vi "Vending_Machine.vi"(0 "Rs100":bool, 1 "Coke":bool, 2 "Fanta":bool, 3 "Sprite":bool, 5 "Rs50":bool, 7 "Rs20":bool, 9 "Rs10":bool, 11 "Rs5":bool, 12 "Cancel":bool, 13 "Open_Door":bool, 14 "Reset":bool) -> (4 "Display_Message":string, 6 "Total_Number_of_Cans":i32 caption="Total Number of Cans", 8 "Total_Cash":i32 caption="Total Cash")   [LabVIEW 2021]
doc: "This is the Coke Vending machine."
uses:
  Controls/Queue_Driver_Select.ctl
  Controls/Inserted_Cash_Count.ctl
  Controls/INI_Operation_Select.ctl
  Controls/Timer_Select.ctl
  Controls/Total_Cash_Count.ctl
  Controls/INI_Data.ctl
  Controls/Controls_Referece.ctl
  Controls/Vending_Data.ctl
panel:
  out "Drink_Ready?":bool
  out "Error_Out":errorcluster
  in  "Error_In":errorcluster
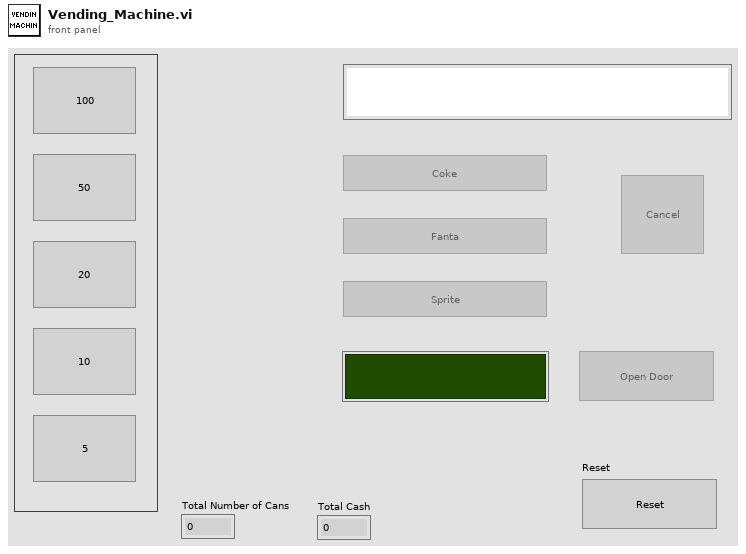
[diagram p1: front panel]
types:
  T1 = typedef "Vending_Data.ctl" = cluster{"INI_Data":T2, "Inserted_Cash_Count":T4, "Drink_Type":string, "Display_Message":string, "Drink_Ready?":bool, "Open_Door":bool, "Cancel":bool, "Reset":bool, "Gray_Out_Control":refnum<vi>[], "Enable_Control":refnum<vi>[], "Disable_Control":refnum<vi>[], "Selected_Cool_Drink":string, "Controls_Reference":T5, "States":string[], "Time_Out":bool, "Exit":bool, "Cost_Per_Can":i32}
  T2 = typedef "INI_Data.ctl" = cluster{"Total_Cash_Count":T3, "Total_Number_of_Cans":i32, "Total_Cash":i32}
  T3 = typedef "Total_Cash_Count.ctl" = cluster{"Rs100":i32, "Rs50":i32, "Rs20":i32, "Rs10":i32, "Rs5":i32}
  T4 = typedef "Inserted_Cash_Count.ctl" = cluster{"Rs100":i32, "Rs50":i32, "Rs20":i32, "Rs10":i32, "Rs5":i32}
  T5 = typedef "Controls_Referece.ctl" = cluster{"Sprite":refnum<vi>, "Fanta":refnum<vi>, "Coke":refnum<vi>, "Cancel":refnum<vi>, "Open_Door":refnum<vi>, "Rs100":refnum<vi>, "Rs50":refnum<vi>, "Rs20":refnum<vi>, "Rs10":refnum<vi>, "Rs5":refnum<vi>, "Reset":refnum<vi>}
  T6 = typedef "INI_Operation_Select.ctl" = enum16{"Read", "Write"}
  T7 = typedef "Queue_Driver_Select.ctl" = enum16{"Obtain_Queue", "Enqueue", "Enqueue_N", "Enqueue_at_Opposite_End", "Preview", "Queue_Status", "Dequeue", "Flush", "Release_Queue"}
  T8 = typedef "Timer_Select.ctl" = enum16{"Start_Timer", "Time_Out?", "Stop_Timer"}
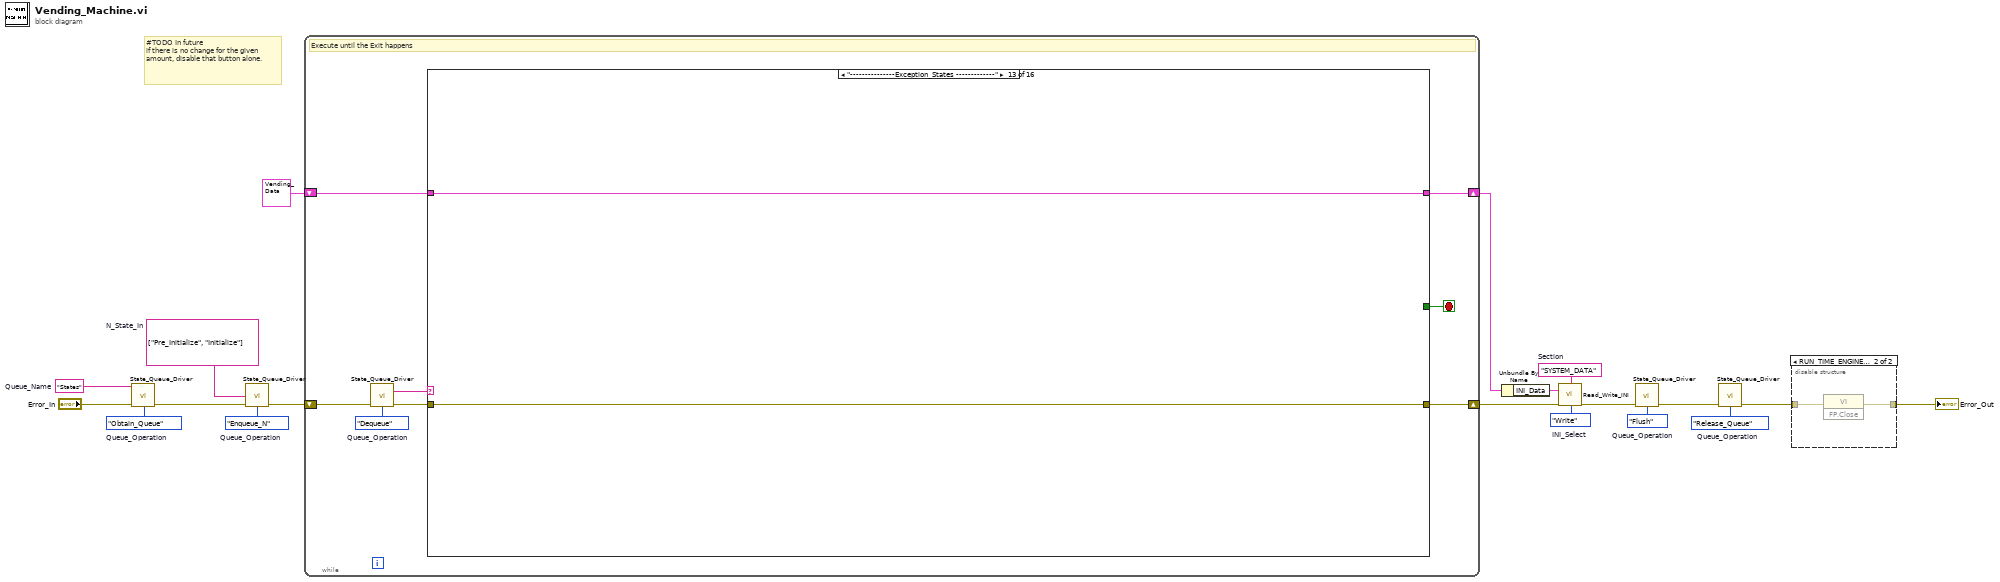
[diagram p0: block diagram]
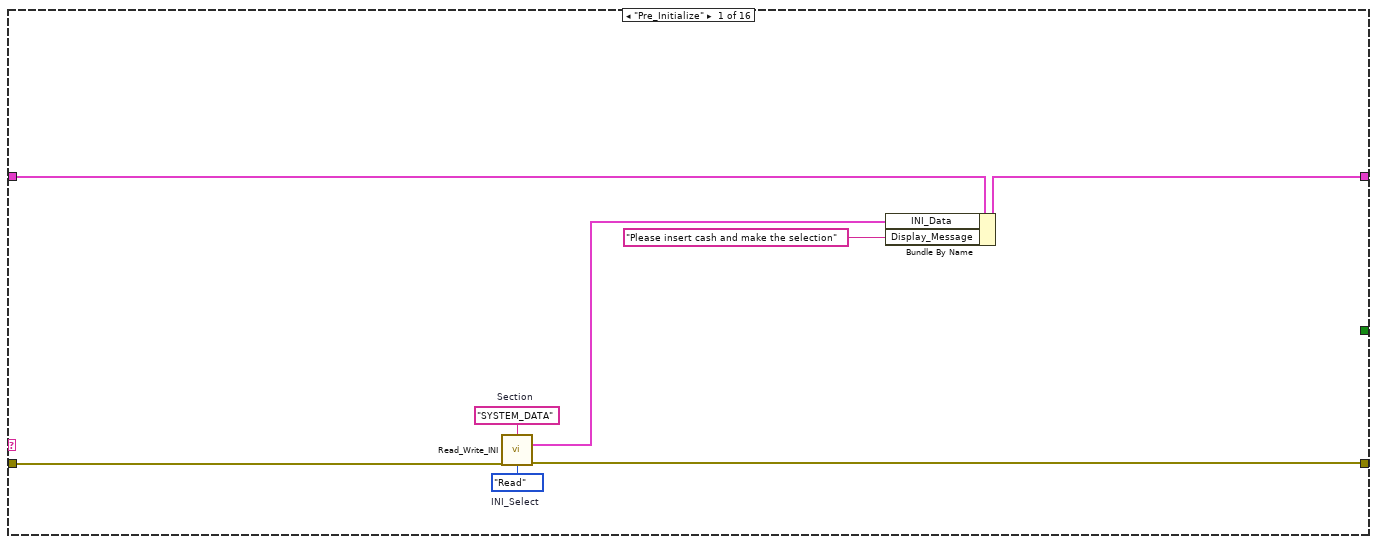
[diagram p2: hidden frame]
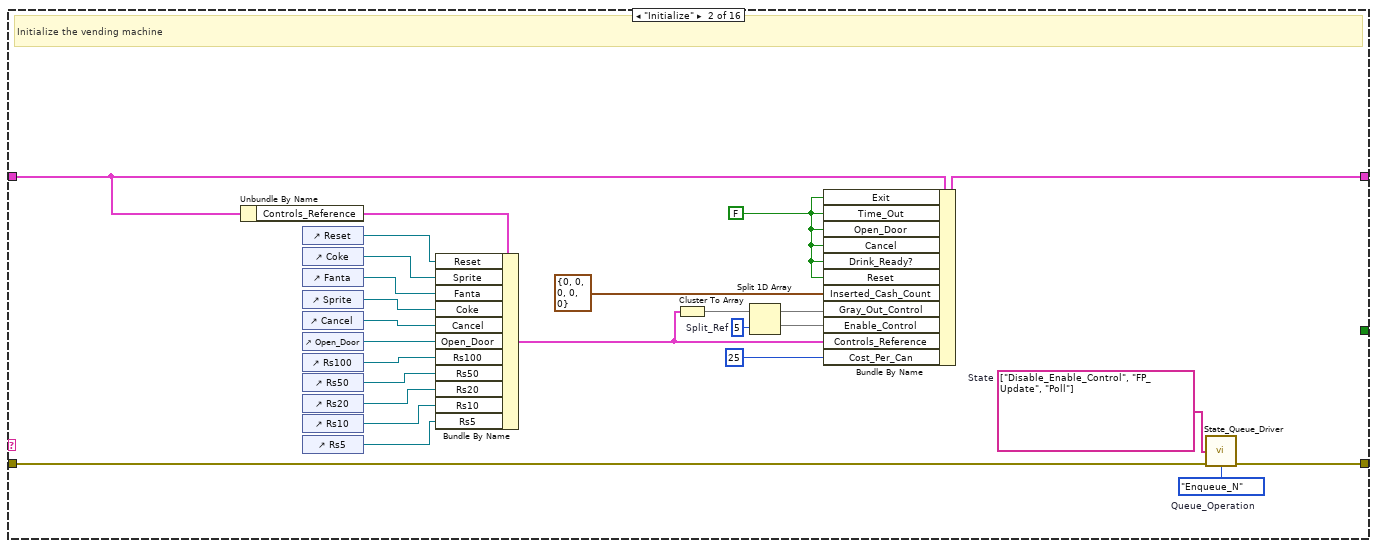
[diagram p3: hidden frame]
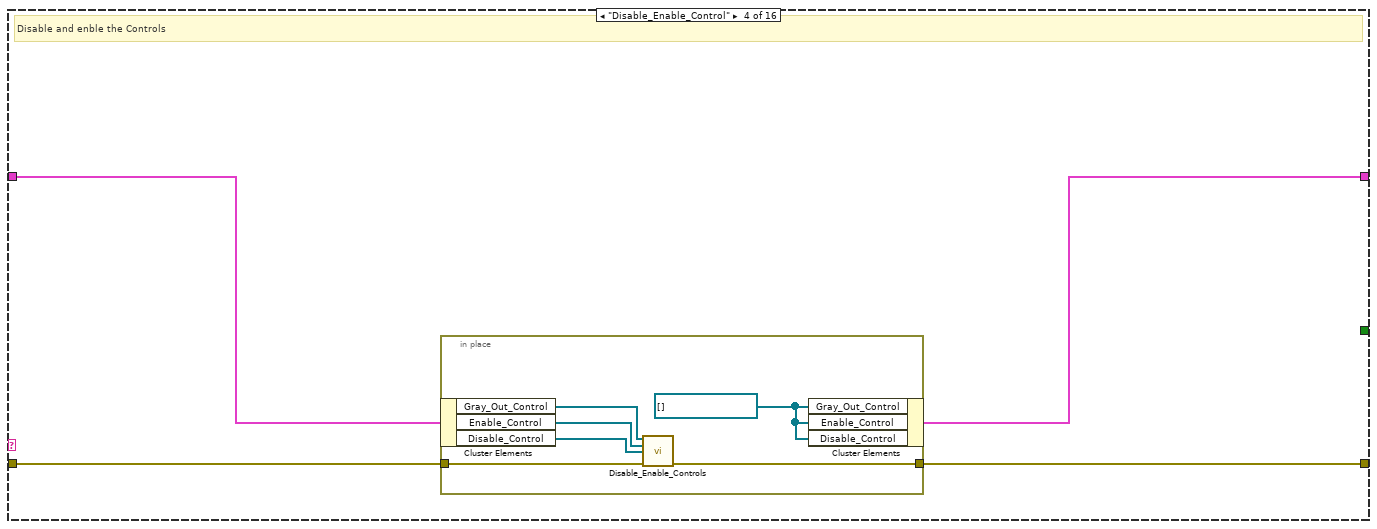
[diagram p5: hidden frame]
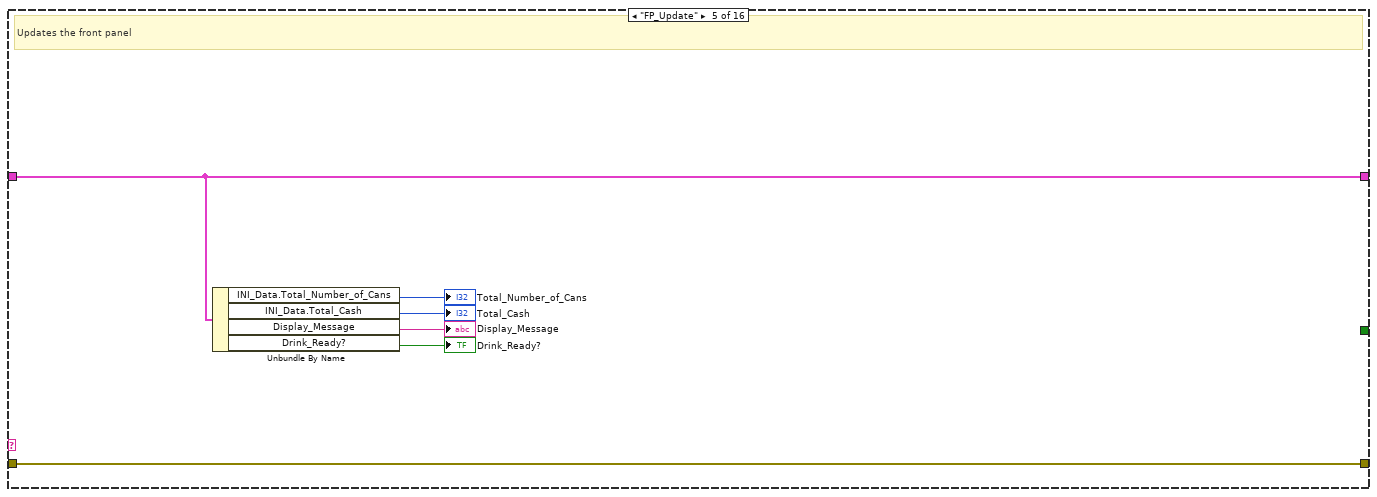
[diagram p6: hidden frame]
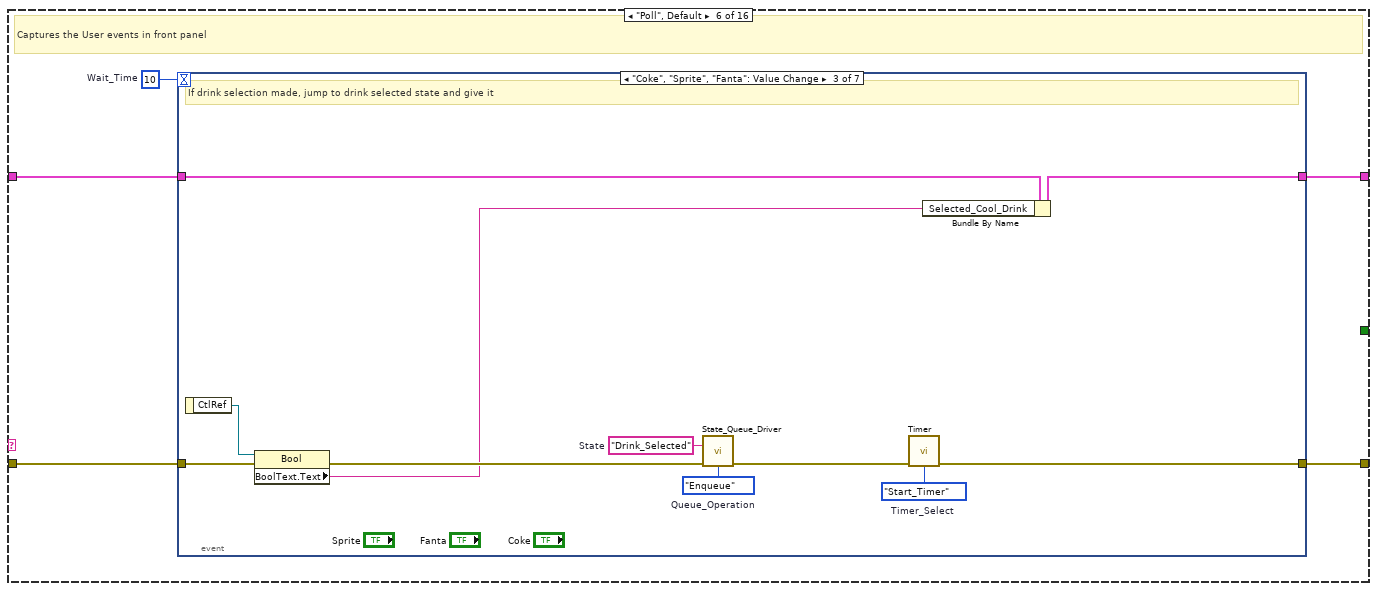
[diagram p7: hidden frame]
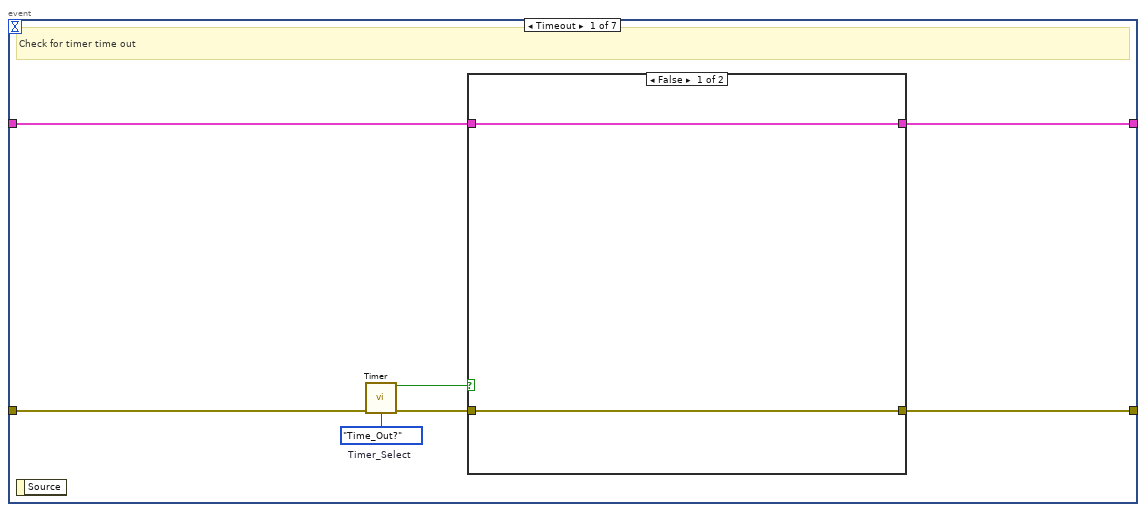
[diagram p8: hidden frame]
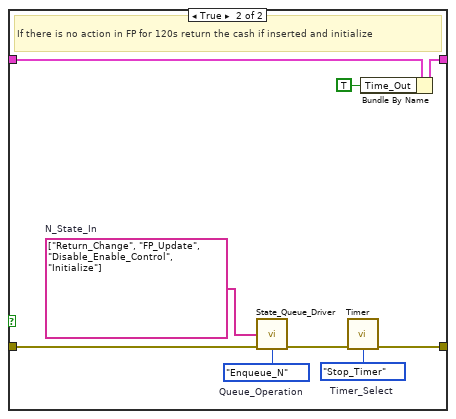
[diagram p9: hidden frame]
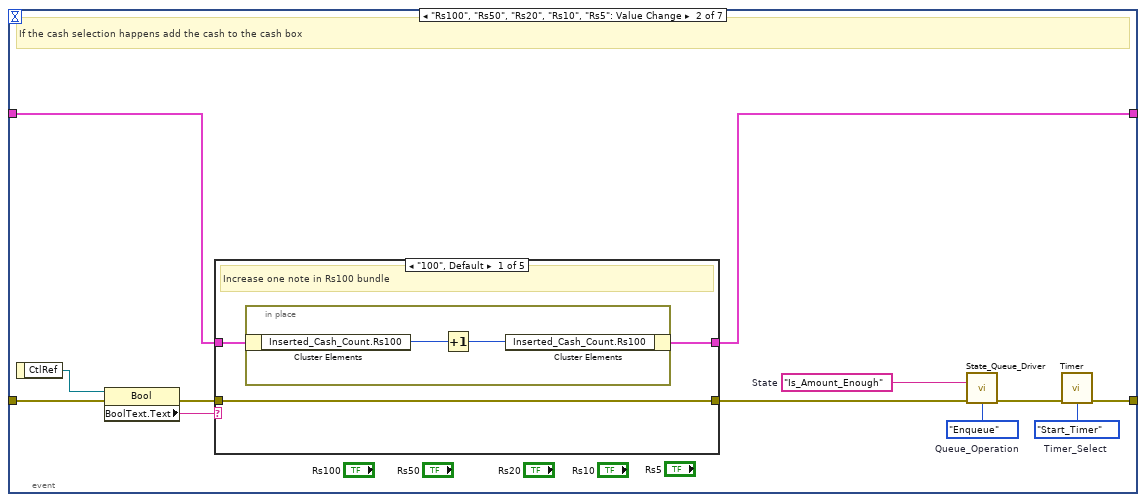
[diagram p10: hidden frame]
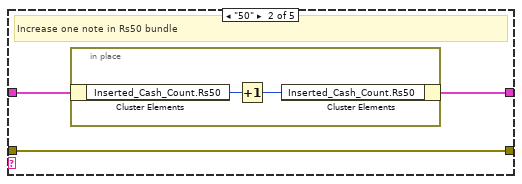
[diagram p11: hidden frame]
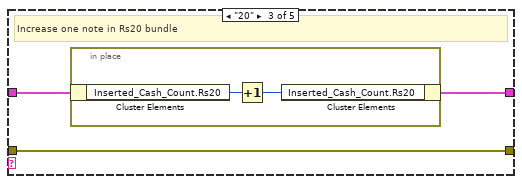
[diagram p12: hidden frame]
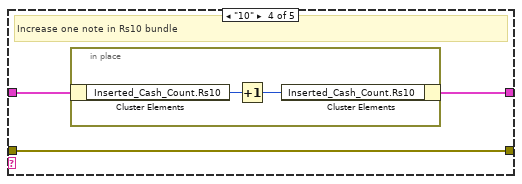
[diagram p13: hidden frame]
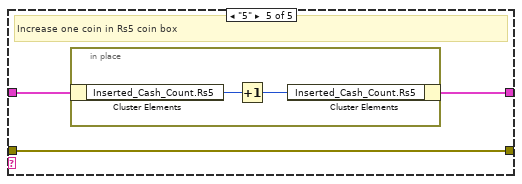
[diagram p14: hidden frame]
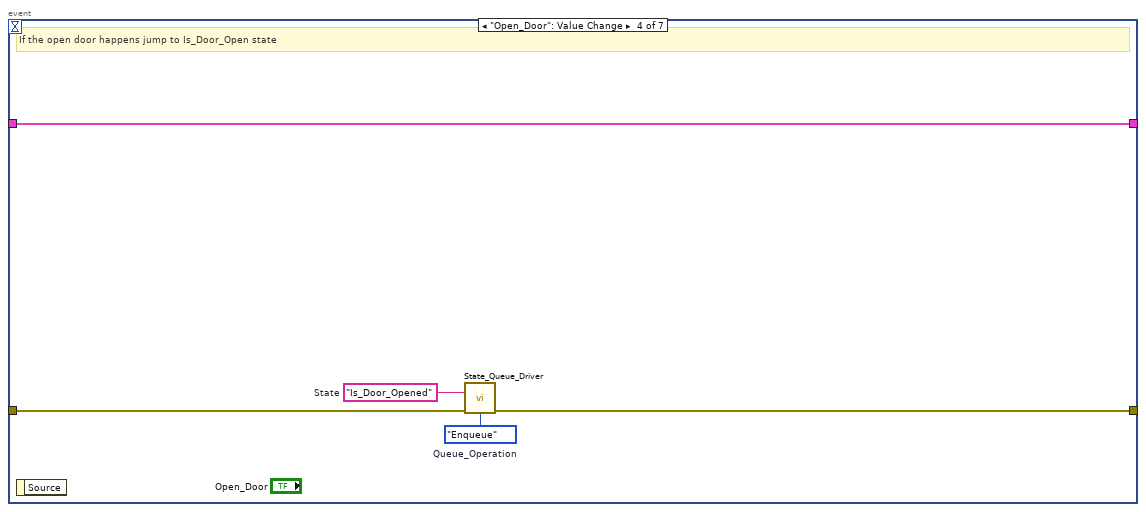
[diagram p15: hidden frame]
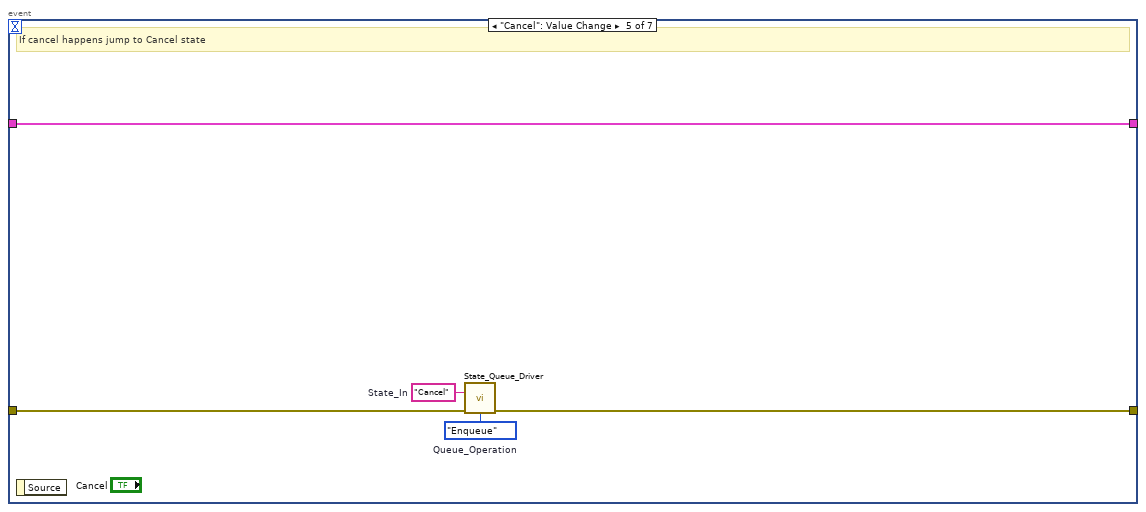
[diagram p16: hidden frame]
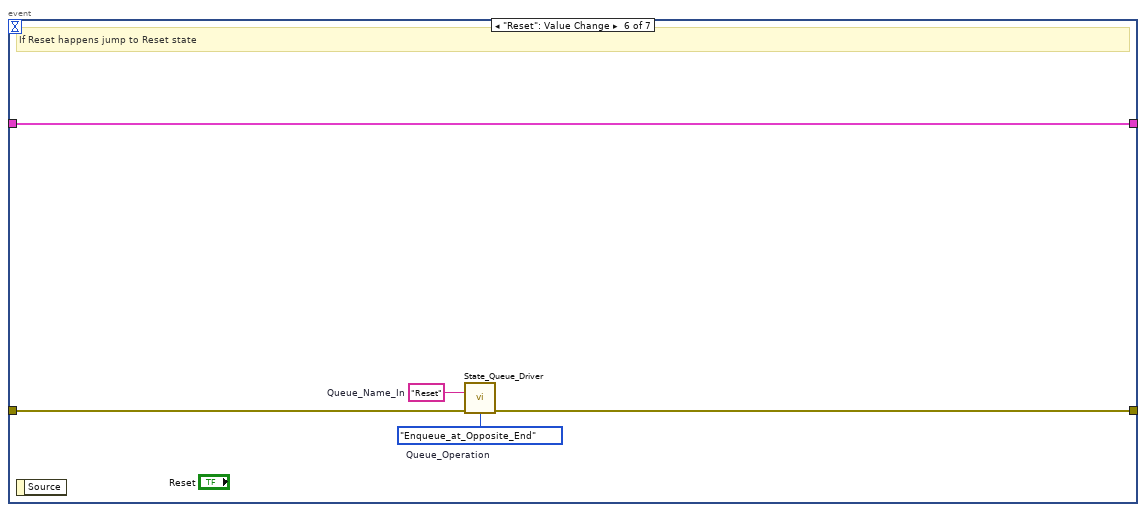
[diagram p17: hidden frame]
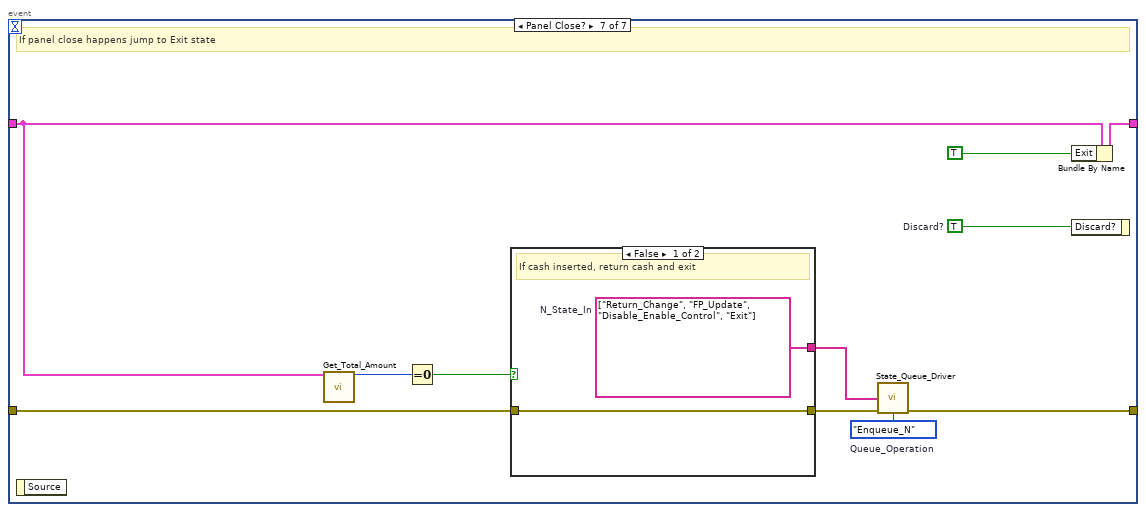
[diagram p18: hidden frame]
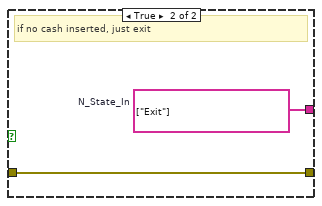
[diagram p19: hidden frame]
diagram:
  w1 = string[] ["Pre_Initialize", "Initialize"]  # N_State_In
  w10 = "SYSTEM_DATA"  # Section
  w9 = INI_Operation_Select."Write"  # INI_Select
  w11 = Queue_Driver_Select."Release_Queue"  # Queue_Operation
  w12 = Queue_Driver_Select."Flush"  # Queue_Operation
  w16 = Queue_Driver_Select."Enqueue_N"  # Queue_Operation
  w17 = "States"  # Queue_Name
  w18 = Queue_Driver_Select."Obtain_Queue"  # Queue_Operation
  # "#TODO In future\nif there is no change for the given amount, disable that button alone."
  n1 = call "State_Queue_Driver.vi"("Queue_Name_In"=w17, "Error_In"="Error_In", "Queue_Operation"=w18) -> ("Error_Out"=w3:errorcluster)  [unwired: 9 in, 3 out]
  n2 = call "State_Queue_Driver.vi"("N_State_In"=w1, "Error_In"=w3, "Queue_Operation"=w16) -> ("Error_Out"=w4:errorcluster)  [unwired: 9 in, 3 out]
  n3 = while {
    shift-right: [w21] -> w7
    shift-left: T1 {"INI_Data"={"Total_Cash_Count"={"Rs100"=0, "Rs50"=0, "Rs20"=0, "Rs10"=0, "Rs5"=0}, "Total_Number_of_Cans"=0, "Total_Cash"=0}, "Inserted_Cash_Count"={"Rs100"=0, "Rs50"=0, "Rs20"=0, "Rs10"=0, "Rs5"=0}, "Drink_Type"="", "Display_Message"="", "Drink_Ready?"=FALSE, "Open_Door"=FALSE, "Cancel"=FALSE, "Reset"=FALSE, "Gray_Out_Control"=[], "Enable_Control"=[], "Disable_Control"=[], "Selected_Cool_Drink"="", "Controls_Reference"={"Sprite"=refnum, "Fanta"=refnum, "Coke"=refnum, "Cancel"=refnum, "Open_Door"=refnum, "Rs100"=refnum, "Rs50"=refnum, "Rs20"=refnum, "Rs10"=refnum, "Rs5"=refnum, "Reset"=refnum}, "States"=[], "Time_Out"=FALSE, "Exit"=FALSE, "Cost_Per_Can"=0} ("Vending_data") -> [w23]
    shift-right: [w20] -> w8
    shift-left: w4 -> [w26]
    stop <- w22 stop-if-true
    w27 = Queue_Driver_Select."Dequeue"  # Queue_Operation
    # "Execute until the Exit happens"
    n4 = call "State_Queue_Driver.vi"("Error_In"=w26, "Queue_Operation"=w27) -> ("State_Out"=w25:string, "Error_Out"=w24:errorcluster)  [unwired: 10 in, 2 out]
    n5 = case shown="\"---------------Exception_States -------------\"" w25 {
      tunnel: [w32 w59 w62 w66 w74 w83 w181 w191 w240 w304 w334 w345 w350 w357 w365 w386] -> w20
      tunnel: w24 -> [w31 w36 w62 w67 w74 w82 w181 w189 w242 w301 w340 w348 w350 w362 w366 w386]
      tunnel: w23 -> [w35 w40 w63 w65 w79 w80 w182 w186 w239 w297 w338 w349 w351 w358 w376 w389]
      tunnel: [w30 w61 w63 w64 w79 w81 w182 w185 w241 w296 w339 w347 w351 w361 w376 w390] -> w21
      tunnel: [_ _ _ _ _ _ _ _ _ _ _ _ _ _ _ w384] -> w22
      frame "Pre_Initialize" {
        w33 = "SYSTEM_DATA"  # Section
        w34 = INI_Operation_Select."Read"  # INI_Select
        n6 = call "Read_Write_INI.vi"("Section"=w33, "Error_In"=w31, "INI_Select"=w34) -> ("Data_Out"=w29:T2, "Error_Out"=w32:errorcluster)  [unwired: 11 in]
        n7 = Bundle By Name(cluster=w35, "INI_Data"=w29, "Display_Message"="Please insert cash and make the selection") -> (w30:T1)
      }
      frame "Initialize" {
        w50 = 5  # Split_Ref
        w58 = Queue_Driver_Select."Enqueue_N"  # Queue_Operation
        w47 = string[] ["Disable_Enable_Control", "FP_Update", "Poll"]  # State
        w41 = FALSE
        # "Initialize the vending machine"
        n8 = Unbundle By Name(w40) -> ("Controls_Reference"=w39:T5)
        n9 = control-ref of="Reset"() -> (w38:refnum<vi>)
        n10 = control-ref of="Coke"() -> (w57:refnum<vi>)
        n11 = control-ref of="Fanta"() -> (w56:refnum<vi>)
        n12 = control-ref of="Sprite"() -> (w55:refnum<vi>)
        n13 = control-ref of="Cancel"() -> (w54:refnum<vi>)
        n14 = control-ref of="Open_Door"() -> (w53:refnum<vi>)
        n15 = control-ref of="Rs100"() -> (w46:refnum<vi>)
        n16 = control-ref of="Rs50"() -> (w45:refnum<vi>)
        n17 = control-ref of="Rs20"() -> (w44:refnum<vi>)
        n18 = control-ref of="Rs10"() -> (w43:refnum<vi>)
        n19 = control-ref of="Rs5"() -> (w42:refnum<vi>)
        n20 = Bundle By Name(cluster=w39, "Reset"=w38, "Sprite"=w57, "Fanta"=w56, "Coke"=w55, "Cancel"=w54, "Open_Door"=w53, "Rs100"=w46, "Rs50"=w45, "Rs20"=w44, "Rs10"=w43, "Rs5"=w42) -> (w52:T5)
        n21 = Cluster To Array(cluster=w52) -> (array=w51:refnum<vi>[])
        n22 = Split 1D Array(array=w51, index=w50) -> (first subarray=w49:refnum<vi>[], second subarray=w48:refnum<vi>[])
        n23 = Bundle By Name(cluster=w40, "Exit"=w41, "Time_Out"=w41, "Open_Door"=w41, "Cancel"=w41, "Drink_Ready?"=w41, "Reset"=w41, "Inserted_Cash_Count"=T4 {"Rs100"=0, "Rs50"=0, "Rs20"=0, "Rs10"=0, "Rs5"=0}, "Gray_Out_Control"=w49, "Enable_Control"=w48, "Controls_Reference"=w52, "Cost_Per_Can"=25) -> (w61:T1)
        n24 = call "State_Queue_Driver.vi"("N_State_In"=w47, "Error_In"=w36, "Queue_Operation"=w58) -> ("Error_Out"=w59:errorcluster)  [unwired: 9 in, 3 out]
      }
      frame "------------User interaction states-----------" {
        # "States after this are user interaction states"
      }
      frame "Disable_Enable_Control" {
        # "Disable and enble the Controls"
        n25 = in-place {
          in-place-border: w67 -> [w73]
          in-place-border: [w71] -> w66
          w68 = refnum<vi>[] [] ("Disable_Control")
          n26 = in-place-cluster #1(w65) -> ("Gray_Out_Control"=w72:refnum<vi>[], "Enable_Control"=w70:refnum<vi>[], "Disable_Control"=w69:refnum<vi>[])
          n27 = call "Disable_Enable_Controls.vi"("Gray_Out_Control"=w72, "Enable_Control"=w70, "Disable_Control"=w69, "Error_In"=w73) -> ("Error_Out"=w71:errorcluster)  [unwired: 11 in]
          n28 = in-place-cluster #1("Gray_Out_Control"=w68, "Enable_Control"=w68, "Disable_Control"=w68) -> (w64:T1)
        }
      }
      frame "FP_Update" {
        # "Updates the front panel"
        n29 = Unbundle By Name(w79) -> ("INI_Data.Total_Number_of_Cans"=→"Total_Number_of_Cans":i32, "INI_Data.Total_Cash"=→"Total_Cash":i32, "Display_Message"=→"Display_Message":string, "Drink_Ready?"=→"Drink_Ready?":bool)
      }
      frame "Poll", Default {
        w84 = 10  # Wait_Time
        # "Captures the User events in front panel"
        n30 = event shown="[2] \"Coke\", \"Sprite\", \"Fanta\": Value Change" {
          selector: _ -> [_ _ _ _ _ _ _]
          dyn-events: _ -> [_ _ _ _ _ _ _]
          timeout: w84 -> [_ _ _ _ _ _ _]
          tunnel: [w87 w106 w141 w153 w158 w164 w175] -> w83
          tunnel: w82 -> [w91 w110 w150 w154 w159 w165 w170]
          tunnel: [w85 w103 w146 w155 w160 w162 w167] -> w81
          tunnel: w80 -> [w86 w114 w147 w155 w160 w162 w173]
          event Timeout {
            w90 = Timer_Select."Time_Out?"  # Timer_Select
            # "Check for timer time out"
            n31 = event-data() -> ()  [unwired: 1 in, 1 out]
            n32 = call "Timer.vi"("Error_In"=w91, "Timer_Select"=w90) -> ("Time_Out?"=w89:bool, "Error_Out"=w88:errorcluster)  [unwired: 12 in]
            n33 = case shown="False" w89 {
              tunnel: w88 -> [w93 w102]
              tunnel: [w93 w98] -> w87
              tunnel: w86 -> [w92 w96]
              tunnel: [w92 w95] -> w85
              frame False {
              }
              frame True {
                w97 = Timer_Select."Stop_Timer"  # Timer_Select
                w99 = string[] ["Return_Change", "FP_Update", "Disable_Enable_Control", "Initialize"]  # N_State_In
                w100 = Queue_Driver_Select."Enqueue_N"  # Queue_Operation
                # "If there is no action in FP for 120s return the cash if inserted and initialize"
                n34 = call "State_Queue_Driver.vi"("N_State_In"=w99, "Error_In"=w102, "Queue_Operation"=w100) -> ("Error_Out"=w101:errorcluster)  [unwired: 9 in, 3 out]
                n35 = call "Timer.vi"("Error_In"=w101, "Timer_Select"=w97) -> ("Error_Out"=w98:errorcluster)  [unwired: 12 in, 1 out]
                n36 = Bundle By Name(cluster=w96, "Time_Out"=TRUE) -> (w95:T1)
              }
            }
          }
          event "Rs100", "Rs50", "Rs20", "Rs10", "Rs5": Value Change {
            w105 = Timer_Select."Start_Timer"  # Timer_Select
            w113 = Queue_Driver_Select."Enqueue"  # Queue_Operation
            w104 = "Is_Amount_Enough"  # State
            # "If the cash selection happens add the cash to the cash box"
            n37 = event-data() -> ("CtlRef"=w108:refnum<vi>)  [unwired: 1 in]
            n38 = property class="Bool"(reference=w108, error in=w110) -> (error out=w109:errorcluster, "BoolText.Text"=w107:string)  [unwired: 1 out]
            n39 = case shown="\"100\", Default" w107 {
              tunnel: w114 -> [w117 w122 w127 w132 w137]
              tunnel: [w116 w121 w126 w131 w136] -> w103
              tunnel: [w115 w120 w125 w130 w135] -> w111
              tunnel: w109 -> [w115 w120 w125 w130 w135]
              frame "100", Default {
                # "Increase one note in Rs100 bundle"
                n40 = in-place {
                  n41 = in-place-cluster #2(w117) -> ("Inserted_Cash_Count.Rs100"=w119:i32)
                  n42 = Increment(x=w119) -> (x+1=w118:i32)
                  n43 = in-place-cluster #2("Inserted_Cash_Count.Rs100"=w118) -> (w116:T1)
                }
              }
              frame "50" {
                # "Increase one note in Rs50 bundle"
                n44 = in-place {
                  n45 = in-place-cluster #3(w122) -> ("Inserted_Cash_Count.Rs50"=w124:i32)
                  n46 = Increment(x=w124) -> (x+1=w123:i32)
                  n47 = in-place-cluster #3("Inserted_Cash_Count.Rs50"=w123) -> (w121:T1)
                }
              }
              frame "20" {
                # "Increase one note in Rs20 bundle"
                n48 = in-place {
                  n49 = in-place-cluster #4(w127) -> ("Inserted_Cash_Count.Rs20"=w129:i32)
                  n50 = Increment(x=w129) -> (x+1=w128:i32)
                  n51 = in-place-cluster #4("Inserted_Cash_Count.Rs20"=w128) -> (w126:T1)
                }
              }
              frame "10" {
                # "Increase one note in Rs10 bundle"
                n52 = in-place {
                  n53 = in-place-cluster #5(w132) -> ("Inserted_Cash_Count.Rs10"=w134:i32)
                  n54 = Increment(x=w134) -> (x+1=w133:i32)
                  n55 = in-place-cluster #5("Inserted_Cash_Count.Rs10"=w133) -> (w131:T1)
                }
              }
              frame "5" {
                # "Increase one coin in Rs5 coin box"
                n56 = in-place {
                  n57 = in-place-cluster #6(w137) -> ("Inserted_Cash_Count.Rs5"=w139:i32)
                  n58 = Increment(x=w139) -> (x+1=w138:i32)
                  n59 = in-place-cluster #6("Inserted_Cash_Count.Rs5"=w138) -> (w136:T1)
                }
              }
            }
            n60 = call "State_Queue_Driver.vi"("State_In"=w104, "Error_In"=w111, "Queue_Operation"=w113) -> ("Error_Out"=w112:errorcluster)  [unwired: 9 in, 3 out]
            n61 = call "Timer.vi"("Error_In"=w112, "Timer_Select"=w105) -> ("Error_Out"=w106:errorcluster)  [unwired: 12 in, 1 out]
          }
          event "Coke", "Sprite", "Fanta": Value Change {
            w140 = Timer_Select."Start_Timer"  # Timer_Select
            w142 = "Drink_Selected"  # State
            w143 = Queue_Driver_Select."Enqueue"  # Queue_Operation
            # "If drink selection made, jump to drink selected state and give it"
            n62 = event-data() -> ("CtlRef"=w149:refnum<vi>)  [unwired: 1 in]
            n63 = property class="Bool"(reference=w149, error in=w150) -> (error out=w148:errorcluster, "BoolText.Text"=w145:string)  [unwired: 1 out]
            n64 = call "State_Queue_Driver.vi"("State_In"=w142, "Error_In"=w148, "Queue_Operation"=w143) -> ("Error_Out"=w144:errorcluster)  [unwired: 9 in, 3 out]
            n65 = call "Timer.vi"("Error_In"=w144, "Timer_Select"=w140) -> ("Error_Out"=w141:errorcluster)  [unwired: 12 in, 1 out]
            n66 = Bundle By Name(cluster=w147, "Selected_Cool_Drink"=w145) -> (w146:T1)
          }
          event "Open_Door": Value Change {
            w151 = Queue_Driver_Select."Enqueue"  # Queue_Operation
            w152 = "Is_Door_Opened"  # State
            # "If the open door happens jump to Is_Door_Open state"
            n67 = event-data() -> ()  [unwired: 1 in, 1 out]
            n68 = call "State_Queue_Driver.vi"("State_In"=w152, "Error_In"=w154, "Queue_Operation"=w151) -> ("Error_Out"=w153:errorcluster)  [unwired: 9 in, 3 out]
          }
          event "Cancel": Value Change {
            w156 = "Cancel"  # State_In
            w157 = Queue_Driver_Select."Enqueue"  # Queue_Operation
            # "If cancel happens jump to Cancel state"
            n69 = event-data() -> ()  [unwired: 1 in, 1 out]
            n70 = call "State_Queue_Driver.vi"("State_In"=w156, "Error_In"=w159, "Queue_Operation"=w157) -> ("Error_Out"=w158:errorcluster)  [unwired: 9 in, 3 out]
          }
          event "Reset": Value Change {
            w161 = "Reset"  # Queue_Name_In
            w163 = Queue_Driver_Select."Enqueue_at_Opposite_End"  # Queue_Operation
            # "If Reset happens jump to Reset state"
            n71 = event-data() -> ()  [unwired: 1 in, 1 out]
            n72 = call "State_Queue_Driver.vi"("State_In"=w161, "Error_In"=w165, "Queue_Operation"=w163) -> ("Error_Out"=w164:errorcluster)  [unwired: 9 in, 3 out]
          }
          event Panel Close? {
            w176 = TRUE  # Discard?
            w174 = Queue_Driver_Select."Enqueue_N"  # Queue_Operation
            # "If panel close happens jump to Exit state"
            n73 = event-data() -> ()  [unwired: 1 in, 1 out]
            n74 = call "Get_Total_Amount.vi"("Vending_data"=w173) -> ("Total_Amount"=w172:i32)  [unwired: 13 in, 1 out]
            n75 = Equal To 0?(x=w172) -> (x = 0?=w168:bool)
            n76 = case shown="False" w168 {
              tunnel: [w177 w180] -> w171
              tunnel: w170 -> [w178 w179]
              tunnel: [w178 w179] -> w169
              frame False {
                w177 = string[] ["Return_Change", "FP_Update", "Disable_Enable_Control", "Exit"]  # N_State_In
                # "If cash inserted, return cash and exit"
              }
              frame True {
                w180 = string[] ["Exit"]  # N_State_In
                # "if no cash inserted, just exit"
              }
            }
            n77 = call "State_Queue_Driver.vi"("N_State_In"=w171, "Error_In"=w169, "Queue_Operation"=w174) -> ("Error_Out"=w175:errorcluster)  [unwired: 9 in, 3 out]
            n78 = Bundle By Name(cluster=w173, "Exit"=TRUE) -> (w167:T1)
            n79 = event-data("Discard?"=w176) -> ()  [unwired: 1 in, 1 out]
          }
        }
      }
      frame "-----Vending_Machine_Process_States-----" {
        # "States after this are vending machine process"
      }
      frame "Is_Amount_Enough" {
        w190 = Queue_Driver_Select."Enqueue_N"  # Queue_Operation
        # "Check if the inserted amount is enough to purchase"
        n80 = call "Get_Total_Amount.vi"("Vending_data"=w186) -> ("Total_Amount"=w184:i32, "Is_Amount_Enough?"=w183:bool)  [unwired: 13 in]
        n81 = case shown="True" w183 {
          tunnel: w189 -> [w203 w233]
          tunnel: [w202 w233] -> w188
          tunnel: [w197 w215] -> w187
          tunnel: w186 -> [w196 w218]
          tunnel: [w204 w232] -> w185
          tunnel: w184 -> [w201 w212]
          frame False {
            w197 = string[] ["Disable_Enable_Control", "FP_Update", "Poll"]  # State_In
            w200 = "Each cool drink costs Rs 25.\nPlease insert the remaining %d to complete your purchase."  # Display_Message
            # "If not enough"
            n82 = Unbundle By Name(w196) -> ("Controls_Reference.Cancel"=w195:refnum<vi>, "Cost_Per_Can"=w192:i32)
            n83 = Subtract(x=w192, y=w201) -> (x-y=w193:i32)
            n84 = Format Into String(format string=w200, initial string="Insufficient Funds\n", error in=w203, w193) -> (resulting string=w198:string, error out=w202:errorcluster)
            n85 = Build Array(w195) -> (w194:refnum<vi>[])
            n86 = Bundle By Name(cluster=w196, "Display_Message"=w198, "Enable_Control"=w194) -> (w204:T1)
          }
          frame True {
            w214 = string[] ["FP_Update", "Return_Change", "Initialize"]  # State_In
            w219 = string[] ["Disable_Enable_Control", "FP_Update", "Poll"]  # State_In
            w229 = "Select the cool drink "  # Display_Message
            # "Check for change & can"
            # "If Enough"
            n87 = Unbundle By Name(w218) -> ("Controls_Reference.Rs100"=w228:refnum<vi>, "Controls_Reference.Rs50"=w227:refnum<vi>, "Controls_Reference.Rs20"=w226:refnum<vi>, "Controls_Reference.Rs10"=w225:refnum<vi>, "Controls_Reference.Rs5"=w224:refnum<vi>, "Controls_Reference.Sprite"=w223:refnum<vi>, "Controls_Reference.Fanta"=w222:refnum<vi>, "Controls_Reference.Coke"=w221:refnum<vi>, "Controls_Reference.Cancel"=w220:refnum<vi>, "INI_Data.Total_Cash_Count"=w213:T3, "Cost_Per_Can"=w208:i32, "INI_Data.Total_Number_of_Cans"=w206:i32)
            n88 = Not Equal To 0?(x=w206) -> (x != 0?=w205:bool)
            n89 = Subtract(x=w212, y=w208) -> (x-y=w211:i32)
            n90 = call "Deduct_Amount.vi"("Total_Cash_Count_In"=w213, "Total_Inserted_Amount"=w211) -> ("Sufficient"=w210:bool)  [unwired: 12 in, 1 out]
            n91 = And(x=w210, y=w205) -> (x .and. y?=w207:bool)
            n92 = Build Array(w228, w227, w226, w225, w224) -> (w231:refnum<vi>[])
            n93 = Build Array(w223, w222, w221, w220) -> (w230:refnum<vi>[])
            n94 = Not(x=w207) -> (.not. x?=w209:bool)
            n95 = Select(t=w229, s=w207, f="No change available" ("Display_Message")) -> (s? t:f=w217:string)
            n96 = Select(t=w219, s=w207, f=w214) -> (s? t:f=w215:string[])
            n97 = Bundle By Name(cluster=w218, "Gray_Out_Control"=w231, "Enable_Control"=w230, "Display_Message"=w217, "Cancel"=w209) -> (w232:T1)
          }
        }
        n98 = call "State_Queue_Driver.vi"("N_State_In"=w187, "Error_In"=w188, "Queue_Operation"=w190) -> ("Error_Out"=w191:errorcluster)  [unwired: 9 in, 3 out]
      }
      frame "Return_Change" {
        # "Return the cash inserted"
        n99 = Unbundle By Name(w239) -> ("Time_Out"=w234:bool, "Exit"=w237:bool, "Cancel"=w236:bool)
        n100 = call "Get_Total_Amount.vi"("Vending_data"=w239) -> ("Total_Amount"=w238:i32)  [unwired: 13 in, 1 out]
        n101 = Compound Arithmetic op=OR(w234, w237, w236) -> (w235:bool)
        n102 = case shown="True" w235 {
          tunnel: w242 -> [w247 w281]
          tunnel: w239 -> [w254 w273]
          tunnel: [w246 w284] -> w241
          tunnel: [w257 w280] -> w240
          tunnel: w238 -> [w256 w276]
          frame False {
            w243 = FALSE  # Inserted_Cash?
            w250 = "\\nPlease take the balance cash of %d"  # Format
            w249 = "Thanks for using me"  # Message
            # "Returns the balance amount"
            n103 = Unbundle By Name(w254) -> ("Cost_Per_Can"=w255:i32)
            n104 = Subtract(x=w256, y=w255) -> (x-y=w253:i32)
            n105 = Format Into String(format string=w250, initial string=w249, error in=w247, w253) -> (resulting string=w251:string, error out=w257:errorcluster)
            n106 = Equal To 0?(x=w253) -> (x = 0?=w252:bool)
            n107 = Select(t=w249, s=w252, f=w251) -> (s? t:f=w248:string)
            n108 = in-place {
              in-place-border: w248 -> [w266]
              in-place-border: w253 -> [w265]
              n109 = in-place-cluster #7(w254) -> ("INI_Data.Total_Cash_Count"=w261:T3, "Inserted_Cash_Count"=w264:T4)  [unwired: 2 out]
              n110 = Coerce To Type(0:w264, 1:w261) -> (2:w263:T3)
              n111 = Add(x=w261, y=w263) -> (x+y=w262:T3)
              n112 = call "Deduct_Amount.vi"("Total_Cash_Count_In"=w262, "Total_Inserted_Amount"=w265) -> ("Total_Cash_Count_Out"=w258:T3)  [unwired: 12 in, 1 out]
              n113 = in-place-cluster #7("INI_Data.Total_Cash_Count"=w258, "Inserted_Cash_Count"=T4 {"Rs100"=0, "Rs50"=0, "Rs20"=0, "Rs10"=0, "Rs5"=0}, "Display_Message"=w266, "Time_Out"=FALSE) -> (w244:T1)
            }
            n114 = call "Get_Total_Amount.vi"("Vending_data"=w244, "Inserted_Cash?"=w243) -> ("Total_Amount"=w245:i32)  [unwired: 12 in, 1 out]
            n115 = Bundle By Name(cluster=w244, "INI_Data.Total_Cash"=w245) -> (w246:T1)
          }
          frame True {
            w274 = "Please insert cash and make the selection"  # Message
            w278 = "\\nCollect your cash Rs%d "  # Format
            w279 = "Oop..! Sorry for the inconvenience"  # Message
            # "Returns the total amount inserted"
            n116 = call "Timer.vi"("Error_In"=w281, "Timer_Select"=Timer_Select."Start_Timer") -> ("Error_Out"=w268:errorcluster)  [unwired: 12 in, 1 out]
            n117 = Unbundle By Name(w273) -> ("Inserted_Cash_Count"=w272:T4)
            n118 = Format Into String(format string=w278, initial string=w279, error in=w268, w276) -> (resulting string=w277:string, error out=w280:errorcluster)
            n119 = Cluster To Array(cluster=w272) -> (array=w271:i32[])
            n120 = Equal To 0?(x=w271) -> (x = 0?=w270:bool[])
            n121 = And Array Elements(Boolean array=w270) -> (logical AND=w269:bool)
            n122 = Select(t=w274, s=w269, f=w277) -> (s? t:f=w275:string)
            n123 = Bundle By Name(cluster=w273, "Inserted_Cash_Count"=T4 {"Rs100"=0, "Rs50"=0, "Rs20"=0, "Rs10"=0, "Rs5"=0}, "Time_Out"=FALSE, "Display_Message"=w275) -> (w284:T1)
          }
        }
      }
      frame "Drink_Selected" {
        w298 = "\\nEnjoy your %s"  # Format
        w299 = "Great Choice"  # Selected_Cool_Drink
        w302 = string[] ["Disable_Enable_Control", "FP_Update", "Poll"]  # State
        w303 = Queue_Driver_Select."Enqueue_N"  # Queue_Operation
        # "Select and confirm the drink"
        n124 = Unbundle By Name(w297) -> ("Controls_Reference.Open_Door"=w291:refnum<vi>, "Controls_Reference.Coke"=w290:refnum<vi>, "Controls_Reference.Fanta"=w289:refnum<vi>, "Controls_Reference.Sprite"=w288:refnum<vi>, "Controls_Reference.Cancel"=w287:refnum<vi>, "Selected_Cool_Drink"=w286:string)
        n125 = Format Into String(format string=w298, initial string=w299, error in=w301, w286) -> (resulting string=w293:string, error out=w300:errorcluster)
        n126 = case shown="\"Sprite\"" w286 {
          tunnel: w289 -> [w313 w315 w331]
          tunnel: w288 -> [w306 w322 w332]
          tunnel: w290 -> [w314 w323 w324]
          tunnel: [w312 w321 w330] -> w305
          tunnel: w300 -> [w312 w321 w330]
          tunnel: [w311 w318 w328] -> w295
          tunnel: [w310 w319 w327] -> w294
          tunnel: w291 -> [w308 w320 w329]
          tunnel: w287 -> [w309 w317 w326]
          tunnel: [w307 w316 w325] -> w285
          frame "Coke", Default {
            # "Disable and grayout the Sprite and fanta"
            n127 = Build Array(w306) -> (w307:refnum<vi>[])
            n128 = Build Array(w308) -> (w311:refnum<vi>[])
            n129 = Build Array(w314, w313, w309) -> (w310:refnum<vi>[])
          }
          frame "Fanta" {
            # "Disable and grayout the coke and Sprite"
            n130 = Build Array(w315) -> (w316:refnum<vi>[])
            n131 = Build Array(w320) -> (w318:refnum<vi>[])
            n132 = Build Array(w323, w322, w317) -> (w319:refnum<vi>[])
          }
          frame "Sprite" {
            # "Disable and grayout the coke and fanta"
            n133 = Build Array(w324) -> (w325:refnum<vi>[])
            n134 = Build Array(w329) -> (w328:refnum<vi>[])
            n135 = Build Array(w331, w332, w326) -> (w327:refnum<vi>[])
          }
        }
        n136 = Bundle By Name(cluster=w297, "Disable_Control"=w285, "Enable_Control"=w295, "Gray_Out_Control"=w294, "Display_Message"=w293, "Drink_Ready?"=TRUE) -> (w296:T1)
        n137 = call "State_Queue_Driver.vi"("N_State_In"=w302, "Error_In"=w305, "Queue_Operation"=w303) -> ("Error_Out"=w304:errorcluster)  [unwired: 9 in, 3 out]
      }
      frame "Is_Door_Opened" {
        w333 = Timer_Select."Start_Timer"  # Timer_Select
        w335 = string[] ["Return_Change", "FP_Update", "Initialize"]  # N_State_In
        w336 = Queue_Driver_Select."Enqueue_N"  # Queue_Operation
        # "Reduce the can"
        n138 = in-place {
          n139 = in-place-cluster #8(w338) -> ("INI_Data.Total_Number_of_Cans"=w342:i32)
          n140 = Decrement(x=w342) -> (x-1=w341:i32)
          n141 = in-place-cluster #8("INI_Data.Total_Number_of_Cans"=w341) -> (w339:T1)
        }
        n142 = call "State_Queue_Driver.vi"("N_State_In"=w335, "Error_In"=w340, "Queue_Operation"=w336) -> ("Error_Out"=w337:errorcluster)  [unwired: 9 in, 3 out]
        n143 = call "Timer.vi"("Error_In"=w337, "Timer_Select"=w333) -> ("Error_Out"=w334:errorcluster)  [unwired: 12 in, 1 out]
      }
      frame "Cancel" {
        w343 = string[] ["Return_Change", "FP_Update", "Initialize"]  # N_State_In
        w344 = Queue_Driver_Select."Enqueue_N"  # Queue_Operation
        # "If cancel return cash and initialize"
        n144 = call "State_Queue_Driver.vi"("N_State_In"=w343, "Error_In"=w348, "Queue_Operation"=w344) -> ("Error_Out"=w345:errorcluster)  [unwired: 9 in, 3 out]
        n145 = Bundle By Name(cluster=w349, "Cancel"=TRUE) -> (w347:T1)
      }
      frame "---------------Exception_States -------------" {
      }
      frame "Reset" {
        w353 = 0 ("Total_Cash_Count.Rs10")
        w355 = "Initialize"  # State
        w356 = Queue_Driver_Select."Enqueue"  # Queue_Operation
        # "Reset the Machine"
        n146 = call "State_Queue_Driver.vi"("State_In"=w355, "Error_In"=w362, "Queue_Operation"=w356) -> ("Error_Out"=w357:errorcluster)  [unwired: 9 in, 3 out]
        n147 = Bundle By Name(cluster=w358, "INI_Data.Total_Number_of_Cans"=100 ("Total_Number_of_Cans"), "INI_Data.Total_Cash"=1000 ("Total_Cash"), "INI_Data.Total_Cash_Count.Rs100"=w353, "INI_Data.Total_Cash_Count.Rs50"=w353, "INI_Data.Total_Cash_Count.Rs20"=w353, "INI_Data.Total_Cash_Count.Rs10"=w353, "INI_Data.Total_Cash_Count.Rs5"=200 ("Total_Cash_Count.Rs5"), "Display_Message"="Please insert cash and make the selection") -> (w361:T1)
      }
      frame "Error_State" {
        w371 = "%d%s%s"  # Format_String
        w372 = "Application Error"  # Initial_String
        w373 = "Stop"  # T_Button
        w374 = "Continue"  # F_Button
        # "If there is error prompt user"
        n148 = call <vilib>:"Clear Errors.vi"("error in (no error)"=w366) -> ("error out"=w369:errorcluster)  [unwired: 5 in, 1 out]
        n149 = Unbundle By Name(w366) -> ("code"=w368:i32, "source"=w367:string)
        n150 = Format Into String(format string=w371, initial string=w372, error in=w369, w368, "\n", w367) -> (resulting string=w375:string, error out=w364:errorcluster)
        n151 = Two Button Dialog(message=w375, 1:w374, 2:w373) -> (T button?=w363:bool)
        n152 = case shown="True" w363 {
          tunnel: [w377 w380] -> w365
          tunnel: w364 -> [w377 w381]
          frame False {
          }
          frame True {
            w378 = "Exit"  # Queue_Name_In
            w379 = Queue_Driver_Select."Enqueue"  # Queue_Operation
            # "Exit the application"
            n153 = call "State_Queue_Driver.vi"("Queue_Name_In"=w378, "Error_In"=w381, "Queue_Operation"=w379) -> ("Error_Out"=w380:errorcluster)  [unwired: 9 in, 3 out]
          }
        }
      }
      frame "Exit" {
        w383 = "No"  # Back
        w382 = "Yes"  # Stop_Execution
        w387 = "Please insert cash and make the selection"  # Display_Message
        # "Exit the application"
        n154 = disable-structure shown="RUN_TIME_ENGINE==True" {
          disable-tunnel: [w391 w392] -> w385
          frame condition #0 (active) {
            w391 = "Do you want to stop the execution"  # Message
            # "Developer mode"
          }
          frame condition #1 {
            w392 = "Do you want to Exit"  # Message
            # "Run time engine mode"
          }
        }
        n155 = Two Button Dialog(message=w385, 1:w383, 2:w382) -> (T button?=w384:bool)
        n156 = Bundle By Name(cluster=w389, "Exit"=FALSE, "Display_Message"=w387) -> (w390:T1)
      }
    }
  }
  n157 = Unbundle By Name(w7) -> ("INI_Data"=w6:T2)
  n158 = call "Read_Write_INI.vi"("Section"=w10, "Data_In"=w6, "Error_In"=w8, "INI_Select"=w9) -> ("Error_Out"=w2:errorcluster)  [unwired: 10 in, 1 out]
  n159 = call "State_Queue_Driver.vi"("Error_In"=w2, "Queue_Operation"=w12) -> ("Error_Out"=w13:errorcluster)  [unwired: 10 in, 3 out]
  n160 = call "State_Queue_Driver.vi"("Error_In"=w13, "Queue_Operation"=w11) -> ("Error_Out"=w14:errorcluster)  [unwired: 10 in, 3 out]
  n161 = disable-structure shown="RUN_TIME_ENGINE==True" {
    disable-tunnel: w14 -> [w393 w395]
    disable-tunnel: [w393 w394] -> w15
    frame condition #0 (active) {
    }
    frame condition #1 {
      n162 = invoke class="VI" method="FP.Close"(error in=w395) -> (error out=w394:errorcluster)  [unwired: 2 in, 2 out]
    }
  }
  "Error_Out" <- w15
